vi "ExecuteButtonAction.vi"(8 "ErrorIn":errorcluster, 9 "WaitForReply":bool, 10 "Command":string, 11 "ObjectIn":refnum<class "ITAFGUIActions.lvclass">) -> (0 "ErrorOut":errorcluster, 3 "ObjectOut":refnum<class "ITAFGUIActions.lvclass">)   [LabVIEW 2021, in "ITAFGUIActions.lvclass"]
uses:
  ITAFGUIActions.lvclass
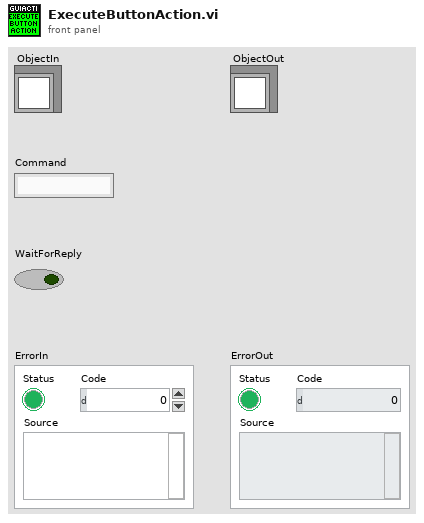
[diagram p1: front panel]
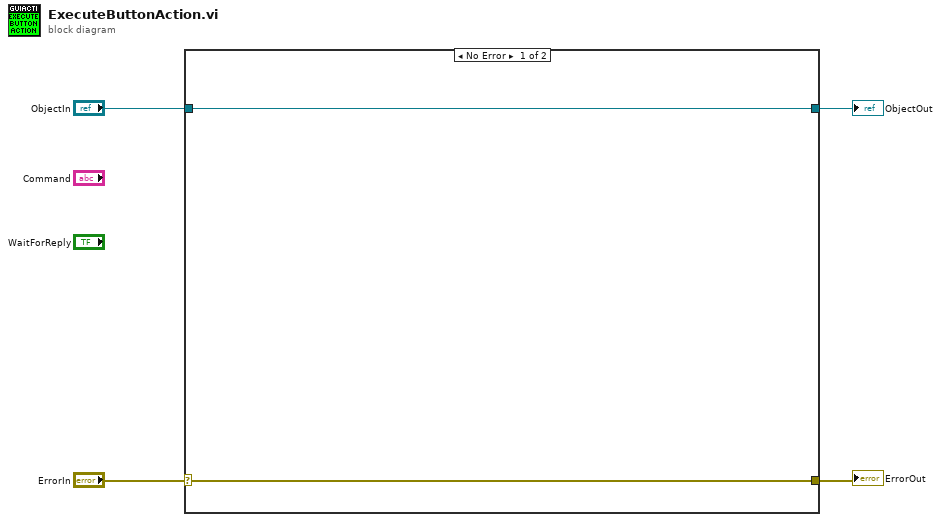
[diagram p0: block diagram]
diagram:
  n1 = case shown="No Error" "ErrorIn" {
    selector: "ErrorIn" -> [w6 w8]
    tunnel: [w6 w8] -> w3
    tunnel: [w5 w7] -> w1
    tunnel: "ObjectIn" -> [w5 w7]
    frame No Error {
    }
    frame Error {
    }
  }
  "ErrorOut" <- w3
  "ObjectOut" <- w1
